vi "get VISA resource name.vi"(8 "error in (no error)":errorcluster caption="Fehler (Eingang, kein Fehler)", 11 "DeviceInterface (Eingang)":refnum<class "DeviceInterface.lvclass">) -> (0 "error out":errorcluster caption="Fehler (Ausgang)", 2 "VISA resource name":refnum<visa-resource-name>, 3 "DeviceInterface (Ausgang)":refnum<class "DeviceInterface.lvclass">)   [LabVIEW 2013, in "DeviceInterface.lvclass"]
uses:
  DeviceInterface.lvclass
  DeviceInterface.lvclass/DeviceInterface.ctl
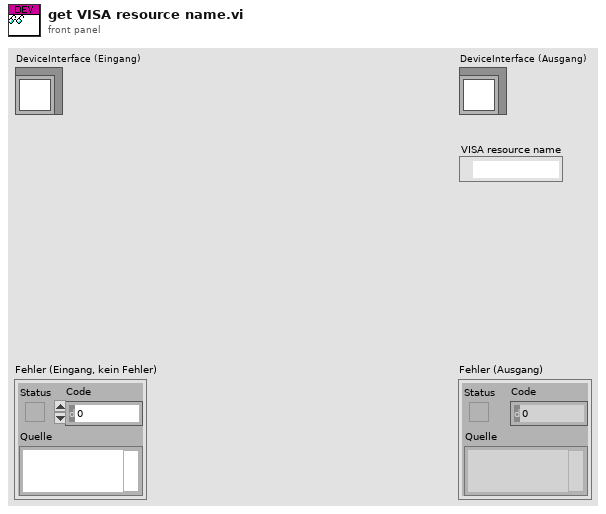
[diagram p1: front panel]
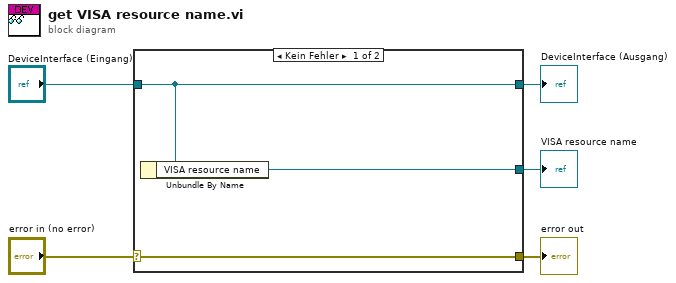
[diagram p0: block diagram]
diagram:
  n1 = case shown="Kein Fehler" "error in (no error)" {
    selector: "error in (no error)" -> [w8 w9]
    tunnel: [w8 w9] -> w4
    tunnel: [w7 w10] -> w2
    tunnel: "DeviceInterface (Eingang)" -> [w7 w10]
    tunnel: [w6 _] -> w1
    frame No Error {
      n2 = Unbundle By Name(w7) -> ("VISA resource name"=w6:refnum<visa-resource-name>)
    }
    frame Error {
    }
  }
  "error out" <- w4
  "DeviceInterface (Ausgang)" <- w2
  "VISA resource name" <- w1
